vi "4Pi Capture File Name Increment.vi"(8 "Step":u16, 9 "Cycle":u16, 10 "laser line":string, 11 "path in":path) -> (3 "path out":path)   [LabVIEW 2016]
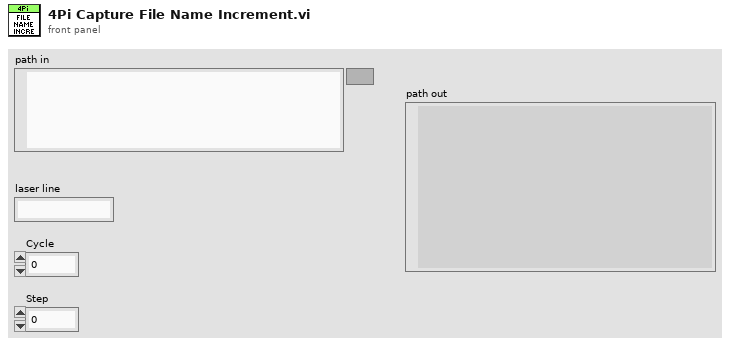
[diagram p1: front panel]
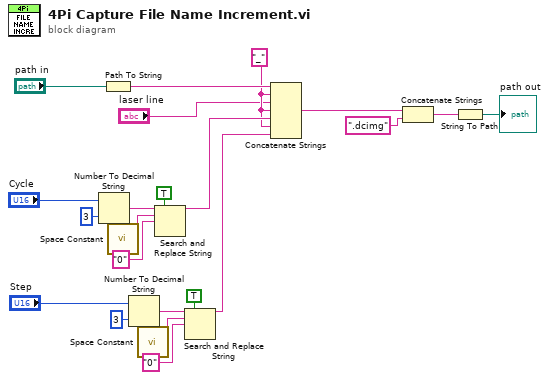
[diagram p0: block diagram]
diagram:
  w10 = "_" ("string")
  n1 = Number To Decimal String(number="Cycle", width (-)=i16 3) -> (decimal integer string=w18:string)
  n2 = Path To String(path="path in") -> (string=w22:string)
  n3 = call <vilib>:"Space Constant.vi"() -> ("String"=w19:string)
  n4 = Number To Decimal String(number="Step", width (-)=i16 3) -> (decimal integer string=w15:string)
  n5 = call <vilib>:"Space Constant.vi"() -> ("String"=w14:string)
  n6 = Search and Replace String(replace all?=TRUE ("replace all? (F)"), input string=w18, search string=w19, replace string="0" ("replace string (\"\")")) -> (result string=w11:string)  [unwired: 4 in, 3 out]
  n7 = Search and Replace String(replace all?=TRUE ("replace all? (F)"), input string=w15, search string=w14, replace string="0" ("replace string (\"\")")) -> (result string=w9:string)  [unwired: 4 in, 3 out]
  n8 = Concatenate Strings(w22, w10, "laser line", w10, w11, w10, w9) -> (w8:string)
  n9 = Concatenate Strings(w8, ".dcimg" ("string")) -> (w7:string)
  n10 = String To Path(string=w7) -> (path=→"path out":path)
